vi "ArrayColorRgbaU64ToImage.vi"(8 "error in":errorcluster, 10 "Pixel":T1[][](array[typedef]), 11 "Image Reference In":T2) -> (0 "error out":errorcluster, 3 "Image Reference Out":T2)   [LabVIEW 2020, in "OpenLvVision_Image.lvlib" / "DataAccess.lvlib"]
doc: "Replaces the image's data with the provided array (Copy)"
uses:
  DataAccess.lvlib
  Management/TypeDef/Image.ctl
  Management/Management.lvlib
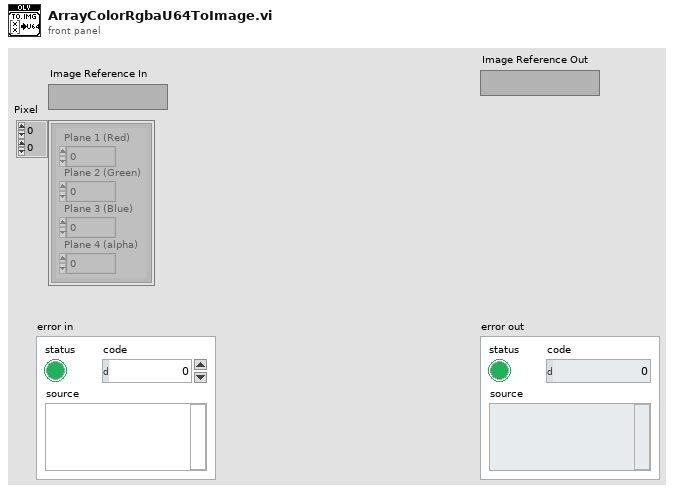
[diagram p1: front panel]
types:
  T1 = typedef "Color (U64)" = cluster{"Plane 3 (Blue)":u16, "Plane 2 (Green)":u16, "Plane 1 (Red)":u16, "Plane 4 (alpha)":u16}
  T2 = typedef "OpenLvVision_Image.lvlib/Management.lvlib/Image.ctl" = refnum<image>
  T3 = typedef "IMAQ Image.ctl" = refnum<image>
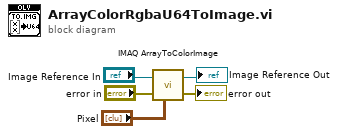
[diagram p0: block diagram]
diagram:
  n1 = call "IMAQ ArrayToColorImage"("Image"="Image Reference In", "Image Pixels (U64)"="Pixel", "error in (no error)"="error in") -> ("Image Out"=→"Image Reference Out":T3, "error out"=→"error out":errorcluster)  [unwired: 2 in]
